vi "异常处理二.vi"() -> ()   [LabVIEW 2023]
panel:
  out "String":string
  out "error out":errorcluster
  # "异常处理 2"
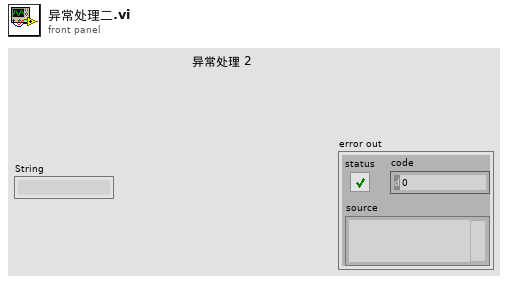
[diagram p1: front panel]
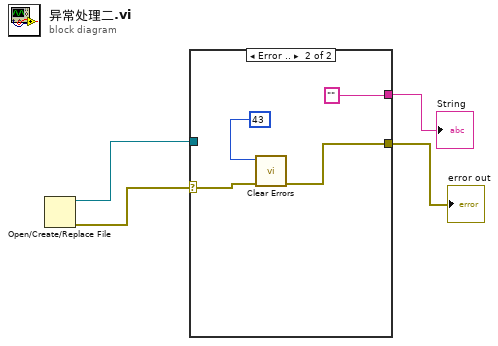
[diagram p0: block diagram]
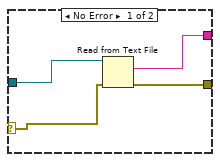
[diagram p2: hidden frame]
diagram:
  n1 = Open/Create/Replace File() -> (refnum out=w3:refnum<file>, error out=w4:errorcluster)  [unwired: 6 in, 1 out]
  n2 = case shown="Error .." w4 {
    selector: w4 -> [w7 w11]
    tunnel: w3 -> [w8 _]
    tunnel: [w6 w10] -> w2
    tunnel: [w5 ""] -> w1
    frame No Error {
      n3 = Read from Text File(file (use dialog)=w8, error in=w7) -> (text=w5:string, error out=w6:errorcluster)  [unwired: 2 in, 2 out]
    }
    frame Error {
      n4 = call <vilib>:"Clear Errors.vi"("error in (no error)"=w11, "specific error code to clear (0: all)"=43) -> ("error out"=w10:errorcluster)  [unwired: 4 in, 1 out]
    }
  }
  "error out" <- w2
  "String" <- w1
